vi "Time Stamp Debug File.vi"(0 "String In":string, 2 "Prepend Stamp":bool) -> (7 "result string":string, 9 "Ends With LF":bool)   [LabVIEW 2014]
panel:
  # "Prepend stamp button indicates that the string initiates a file record and\nrequires a leading time stamp. All linefeeds (\\n) are replaced with \\n time stamp\nunless the string ends with \\n. In that case, the trailing \\n is not given a time stamp\nand the Ends With LF output is 1, indicating that a prepend is required for the\nnext record."
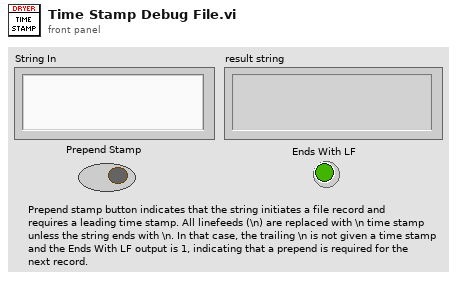
[diagram p1: front panel]
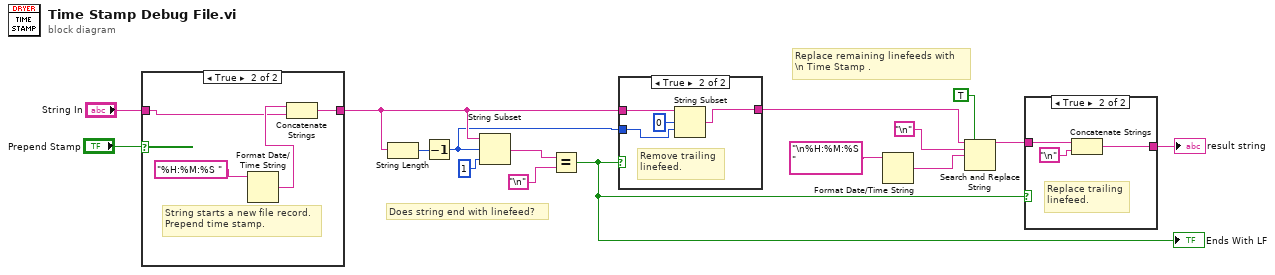
[diagram p0: block diagram]
diagram:
  # "Does string end with linefeed?"
  # "Replace remaining linefeeds with\n\\n Time Stamp ."
  n1 = case shown="True" "Prepend Stamp" {
    tunnel: "String In" -> [w17 w18]
    tunnel: [w17 w21] -> w7
    frame False {
      # "String is not at the beginning\nof the file record.\nDo not prepens time stamp."
    }
    frame True {
      # "String starts a new file record.\nPrepend time stamp."
      n2 = Format Date/Time String(time format string (%c)="%H:%M:%S ") -> (date/time string=w19:string)  [unwired: 2 in]
      n3 = Concatenate Strings(w19, w18) -> (w21:string)
    }
  }
  n4 = String Length(string=w7) -> (length=w10:i32)
  n5 = Decrement(x=w10) -> (x-1=w5:i32)
  n6 = String Subset(string=w7, offset (0)=w5, length (rest)=1 ("length (rest)")) -> (substring=w8:string)
  n7 = Equal?(x=w8, y="\n") -> (x = y?=w4:bool)
  "Ends With LF" <- w4
  n8 = case shown="True" w4 {
    tunnel: w7 -> [w22 w26]
    tunnel: [w22 w23] -> w6
    tunnel: w5 -> [_ w24]
    frame False {
      # "Does not end in LF.\nDo nothing."
    }
    frame True {
      # "Remove trailing\nlinefeed."
      n9 = String Subset(string=w26, offset (0)=0, length (rest)=w24) -> (substring=w23:string)
    }
  }
  n10 = Format Date/Time String(time format string (%c)="\n%H:%M:%S ") -> (date/time string=w15:string)  [unwired: 2 in]
  n11 = Search and Replace String(replace all?=TRUE ("replace all? (F)"), input string=w6, search string="\n", replace string=w15) -> (result string=w3:string)  [unwired: 4 in, 3 out]
  n12 = case shown="True" w4 {
    tunnel: w3 -> [w27 w30]
    tunnel: [w27 w28] -> w2
    frame False {
      # "No trailing linefeed.\nDo nothing."
    }
    frame True {
      # "Replace trailing\nlinefeed."
      n13 = Concatenate Strings(w30, "\n") -> (w28:string)
    }
  }
  "result string" <- w2
